vi "Stop Core.vi"(10 "final error code":i32 caption="最终错误代码", 11 "Log in":refnum<class "Log.lvclass"> caption="操作者输入") -> (3 "Log out":refnum<class "Log.lvclass"> caption="操作者输出")   [LabVIEW 2018, in "Log.lvlib" / "Log.lvclass"]
doc: "(<B>文件名</B>: Actor Framework.lvlib:Actor.lvclass:Stop Core.vi)\n\n定义停止前操作者的动作。Use the <B>final error code</B> input to determine whether the actor shut down in response to an error.\n\nBy default, this method passes the Stop message along to all auto-stop nested actors.A descendant class may override this method to define additional behavior, such as shutting down any processes the actor initiated in its override of the Actor Core method."
uses:
  Log.lvclass
  <vilib>/ActorFramework/Actor/Actor.lvclass
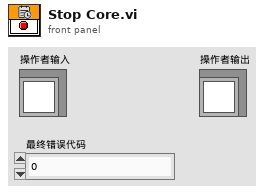
[diagram p1: front panel]
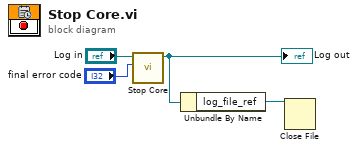
[diagram p0: block diagram]
diagram:
  n1 = call-parent "Stop Core.vi"("final error code"="final error code", "Actor in"="Log in") -> ("Actor out"=w2:refnum<class "Log.lvclass">)  [unwired: 9 in]
  "Log out" <- w2
  n2 = Unbundle By Name(w2) -> ("log_file_ref"=w1:refnum<file>)
  n3 = Close File(refnum=w1) -> ()  [unwired: 1 in, 2 out]
